vi "SettingButton_MenuActive.vi"(8 "error in":errorcluster caption="错误输入（无错误）", 10 "Menu Ref":refnum<k9>, 11 "PCM PanelSplit in":refnum<class "PCM PanelSplit.lvclass"> caption="DNL_LabVIEW Object in") -> (0 "error out":errorcluster caption="错误输出", 3 "PCM PanelSplit out":refnum<class "PCM PanelSplit.lvclass"> caption="DNL_LabVIEW Object out")   [LabVIEW 2016, in "PCM PanelSplit.lvclass"]
uses:
  PCM PanelSplit.lvclass
  Display Mode.ctl
  <vilib>/Analysis/4window.llb/windowTd.ctl
  DAQ-Config/SubVIs/FGV_Cards.ctl
  GlobleVariables/Ctrl_Sample Configure.ctl
  <vilib>/Analysis/NI_AALPro.lvlib
panel:
  in  "window":T1 caption="窗" items=["Rectangle"=0, "Hanning"=1, "Hamming"=2, "Blackman-Harris"=3, "Exact Blackman"=4, "Blackman"=5, "Flat Top"=6, "4 Term B-Harris "=7, "7 Term B-Harris"=8, "Low Sidelobe"=9, "Blackman Nuttall"=11, "Triangle"=30, "Bartlett-Hanning"=31, "Bohman"=32, "Parzen"=33, "Welch"=34, "Kaiser"=60, "Dolph-Chebyshev"=61, "Gaussian"=62]
  in  "Display Mode":T2
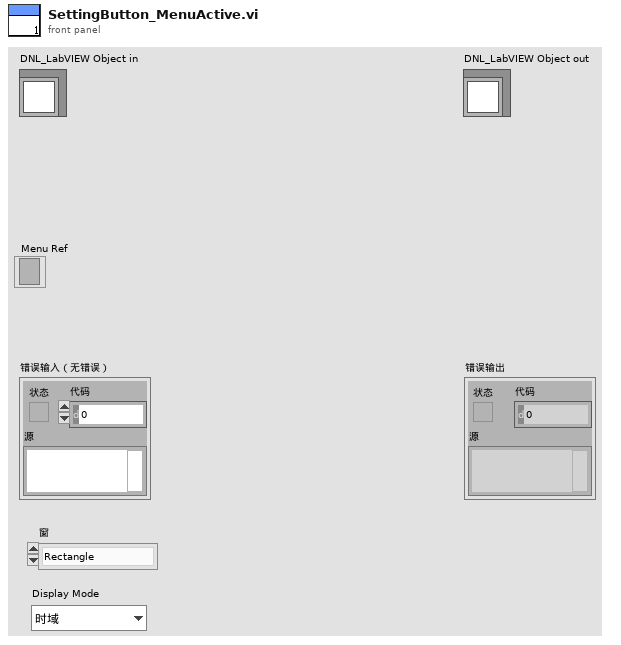
[diagram p1: front panel]
types:
  T1 = typedef "NI_AALPro.lvlib/windowTd.ctl" = u32
  T2 = typedef "PCM PanelSplit.lvclass/Display Mode.ctl" = enum16{"时域", "频谱", "功率谱"}
  T3 = typedef "Ctrl_Sample Configure.ctl" = enum16{"Read", "Set"}
  T4 = typedef "FGV_Cards.ctl" = enum16{"Initlize", "Set_DAQCards", "Set_VCHCards", "Get_DAQCards", "Get_VCHCards", "Get_ALLUsing"}
  T5 = typedef "PCM PanelSplit.lvclass/Display Config.ctl" = cluster{"Display Mode":T2, "ChTag[]":string[], "window":T1, "Range":T6}
  T6 = typedef "LVRangeTypeDef.ctl" = cluster{"Minimum":dbl, "Maximum":dbl, "Increment":dbl, "Minor Increment":dbl, "Start":dbl}
  T7 = cluster{"SignalType":string[], "Channels Tag":string[], "Channels Name":string[], "Unit":string[], "Alarm Upper Limit":dbl[], "Alarm Lower Limit":dbl[], "Sensitivity":dbl[], "SampleRate":dbl[], "Sensor":string[]}
  T8 = typedef "PSCHN_Card Para.ctl" = cluster{"Module Type":string, "Module Name":string, "ModuSN":string, "ModuIP":string, "Used?":bool, "Connected":bool, "Timing*":cluster{"Sample Rate":dbl}, "Channels":T9[]}
  T9 = typedef "PSCHN_Channel Para.ctl" = cluster{"CHTag*":string, "Used?*":bool, "CHName":string, "Unit":string, "斜率":dbl, "截距":dbl}
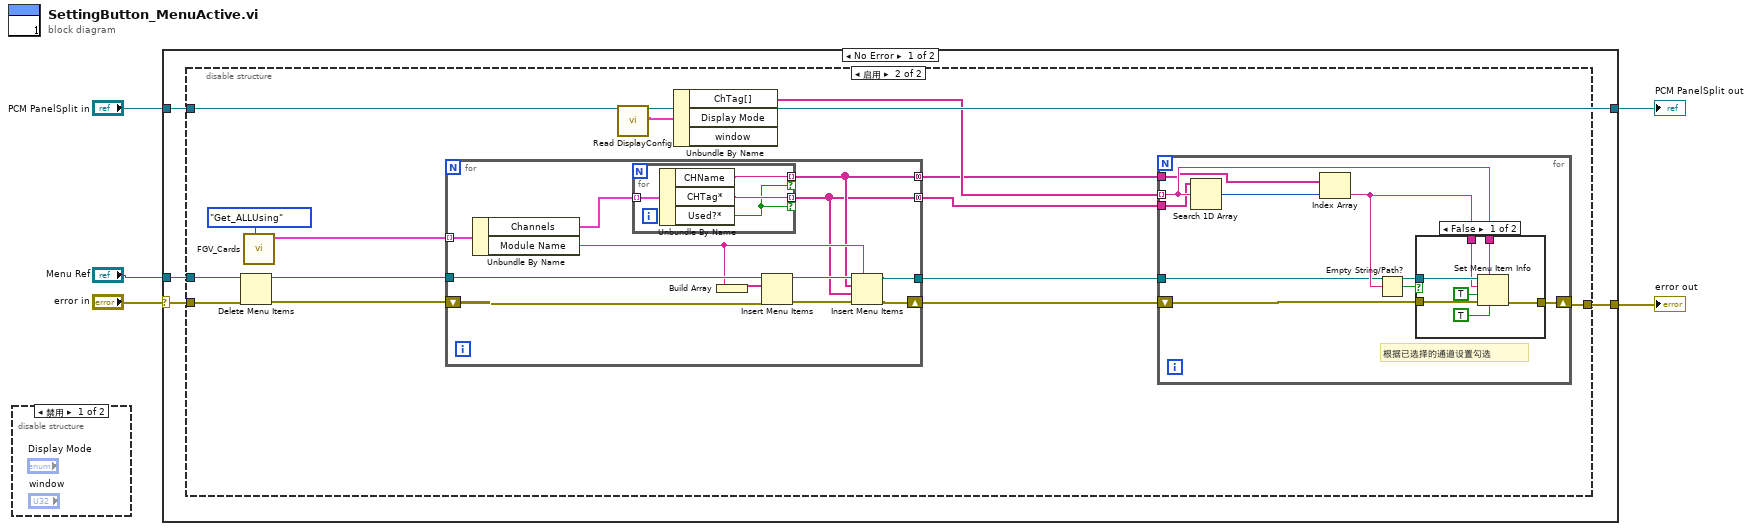
[diagram p0: block diagram]
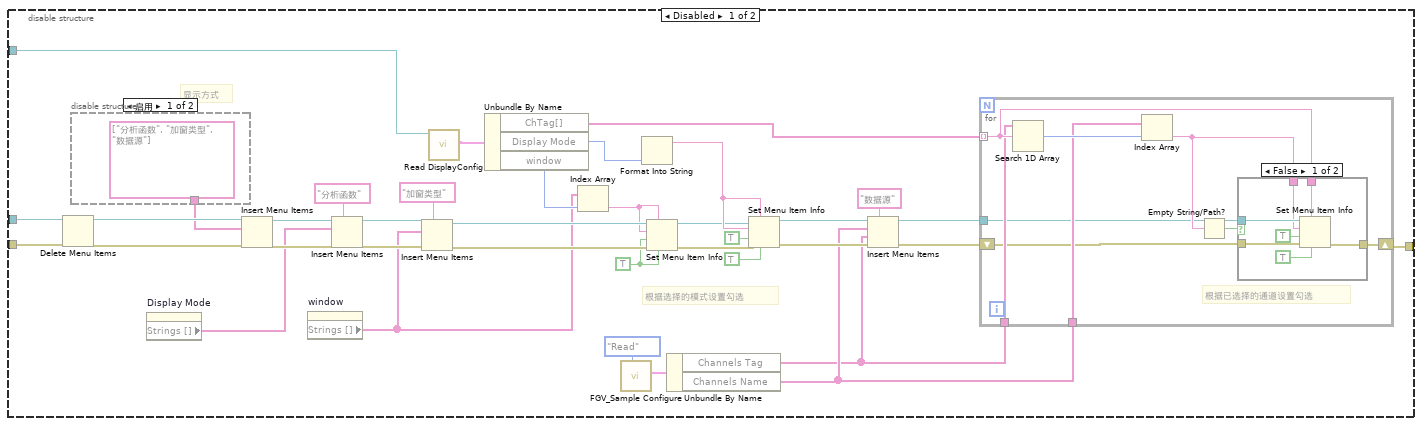
[diagram p3: hidden frame]
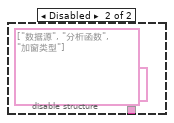
[diagram p5: hidden frame]
diagram:
  n1 = disable-structure shown="禁用" {
    frame Disabled {
    }
    frame Enabled {
    }
  }
  n2 = case shown="No Error" "error in" {
    selector: "error in" -> [w9 w113]
    tunnel: [w8 w113] -> w1
    tunnel: [w6 w114] -> w3
    tunnel: "PCM PanelSplit in" -> [w6 w114]
    tunnel: "Menu Ref" -> [w7 _]
    frame No Error {
      n3 = disable-structure shown="启用" {
        disable-tunnel: w9 -> [w38 w79]
        disable-tunnel: [w37 w78] -> w8
        disable-tunnel: w7 -> [w36 w77]
        disable-tunnel: w6 -> [w35 w76]
        frame Disabled {
          w25 = TRUE ("已勾选")
          # "显示方式"
          # "根据选择的模式设置勾选"
          n4 = Delete Menu Items(6:w38, 9:w36) -> (0:w45:errorcluster, 3:w46:refnum<k9>)  [unwired: 2 in]
          n5 = disable-structure shown="启用" {
            disable-tunnel: [string[] ["分析函数", "加窗类型", "数据源"] ("项名称") string[] ["数据源", "分析函数", "加窗类型"] ("项名称")] -> w42
            frame Enabled {
            }
            frame Disabled {
            }
          }
          n6 = property on="Display Mode" class="Enum (strict)"() -> ("Strings []"=w33:string[])  [unwired: 2 in, 2 out]
          n7 = Insert Menu Items(6:w45, 8:w42, 9:w46) -> (0:w44:errorcluster, 3:w43:refnum<k9>)  [unwired: 3 in, 1 out]
          n8 = property on="window" class="Ring (strict)"() -> ("Strings []"=w21:string[])  [unwired: 2 in, 2 out]
          n9 = Insert Menu Items(5:"分析函数", 6:w44, 8:w33, 9:w43) -> (0:w29:errorcluster, 3:w30:refnum<k9>)  [unwired: 2 in, 1 out]
          n10 = Insert Menu Items(5:"加窗类型" ("菜单标识符"), 6:w29, 8:w21, 9:w30) -> (0:w27:errorcluster, 3:w23:refnum<k9>)  [unwired: 2 in, 1 out]
          n11 = call "Read DisplayConfig.vi"("PCM PanelSplit 输入"=w35) -> ("Display Config"=w34:T5)  [unwired: 8 in, 2 out]
          n12 = Unbundle By Name(w34) -> ("ChTag[]"=w17:string[], "Display Mode"=w32:T2, "window"=w22:T1)
          n13 = Index Array(array=w21, index=w22) -> (element=w20:string)
          n14 = call "FGV_Sample Configure.vi"("Action"=Ctrl_Sample_Configure."Read") -> ("SignalTable"=w19:T7)  [unwired: 9 in, 1 out]
          n15 = Format Into String(w32) -> (resulting string=w31:string)  [unwired: 3 in, 1 out]
          n16 = Set Menu Item Info(6:w25, 7:w20, 8:w27, 9:w25, 10:w20, 11:w23) -> (0:w26:errorcluster, 3:w24:refnum<k9>)  [unwired: 1 in]
          n17 = Unbundle By Name(w19) -> ("Channels Tag"=w10:string[], "Channels Name"=w11:string[])
          n18 = Set Menu Item Info(6:TRUE ("已勾选"), 7:w31, 8:w26, 9:TRUE ("已启用"), 10:w31, 11:w24) -> (0:w12:errorcluster, 3:w15:refnum<k9>)  [unwired: 1 in]
          n19 = Insert Menu Items(5:"数据源", 6:w12, 7:w10, 8:w11, 9:w15) -> (0:w13:errorcluster, 3:w14:refnum<k9>)  [unwired: 1 in, 1 out]
          n20 = for {
            tunnel: w14 -> [w48]
            tunnel: w17 -> [w51] mode=indexing
            tunnel: w10 -> [w50]
            tunnel: w11 -> [w49]
            shift-right: [w55] -> w37
            shift-left: w13 -> [w47]
            # "根据已选择的通道设置勾选"
            n21 = Search 1D Array(1D array=w50, element=w51) -> (index of element=w54:i32)  [unwired: 1 in]
            n22 = Index Array(array=w49, index=w54) -> (element=w52:string)
            n23 = Empty String/Path?(string/path=w52) -> (empty?=w53:bool)
            n24 = case shown="False" w53 {
              tunnel: w47 -> [w60 w63]
              tunnel: w48 -> [w59 _]
              tunnel: [w58 w63] -> w55
              tunnel: w52 -> [w57 _]
              tunnel: w51 -> [w56 _]
              frame False {
                n25 = Set Menu Item Info(6:TRUE ("已勾选"), 7:w56, 8:w60, 9:TRUE ("已启用"), 10:w57, 11:w59) -> (0:w58:errorcluster)  [unwired: 1 in, 1 out]
              }
              frame True {
              }
            }
          }
        }
        frame Enabled {
          n26 = Delete Menu Items(6:w79, 9:w77) -> (0:w68:errorcluster, 3:w69:refnum<k9>)  [unwired: 2 in]
          n27 = call "FGV_Cards.vi"("Action"=FGV_Cards."Get_ALLUsing") -> ("Cards out"=w67:T8[])  [unwired: 9 in, 1 out]
          n28 = for {
            tunnel: w69 -> [w91]
            tunnel: w67 -> [w89] mode=indexing
            shift-right: [w85] -> w73
            shift-left: w68 -> [w90]
            tunnel: [w84] -> w72
            tunnel: [w82] -> w70 mode=concatenating
            tunnel: [w81] -> w71 mode=concatenating
            n29 = Unbundle By Name(w89) -> ("Channels"=w83:T9[], "Module Name"=w86:string)
            n30 = for {
              tunnel: w83 -> [w95] mode=indexing
              tunnel: [w94] -> w81 mode=indexing if=w92
              tunnel: [w93] -> w82 mode=indexing if=w92
              n31 = Unbundle By Name(w95) -> ("CHName"=w93:string, "CHTag*"=w94:string, "Used?*"=w92:bool)
            }
            n32 = Build Array(w86) -> (w80:string[])
            n33 = Insert Menu Items(6:w90, 8:w80, 9:w91) -> (0:w87:errorcluster, 3:w88:refnum<k9>)  [unwired: 3 in, 1 out]
            n34 = Insert Menu Items(5:w86, 6:w87, 7:w81, 8:w82, 9:w88) -> (0:w85:errorcluster, 3:w84:refnum<k9>)  [unwired: 1 in, 1 out]
          }
          n35 = call "Read DisplayConfig.vi"("PCM PanelSplit 输入"=w76) -> ("Display Config"=w75:T5)  [unwired: 8 in, 2 out]
          n36 = Unbundle By Name(w75) -> ("ChTag[]"=w74:string[])  [unwired: 2 out]
          n37 = for {
            tunnel: w72 -> [w99]
            tunnel: w74 -> [w101] mode=indexing
            tunnel: w71 -> [w100]
            shift-right: [w104] -> w78
            shift-left: w73 -> [w98]
            tunnel: w70 -> [w97]
            # "根据已选择的通道设置勾选"
            n38 = Search 1D Array(1D array=w100, element=w101) -> (index of element=w103:i32)  [unwired: 1 in]
            n39 = Index Array(array=w97, index=w103) -> (element=w102:string)
            n40 = Empty String/Path?(string/path=w102) -> (empty?=w96:bool)
            n41 = case shown="False" w96 {
              tunnel: w98 -> [w109 w112]
              tunnel: w99 -> [w108 _]
              tunnel: [w107 w112] -> w104
              tunnel: w102 -> [w106 _]
              tunnel: w101 -> [w105 _]
              frame False {
                n42 = Set Menu Item Info(6:TRUE ("已勾选"), 7:w105, 8:w109, 9:TRUE ("已启用"), 10:w106, 11:w108) -> (0:w107:errorcluster)  [unwired: 1 in, 1 out]
              }
              frame True {
              }
            }
          }
        }
      }
    }
    frame Error {
    }
  }
  "error out" <- w1
  "PCM PanelSplit out" <- w3
